vi "Get U16 Data.vi"(8 "error in (no error)":errorcluster, 11 "Data in":string) -> (0 "error out":errorcluster, 2 "U16":u16, 3 "Data out":string)   [LabVIEW 2013, in "Hierarchy Framework.lvlib" / "Section.lvclass"]
uses:
  Section.lvclass
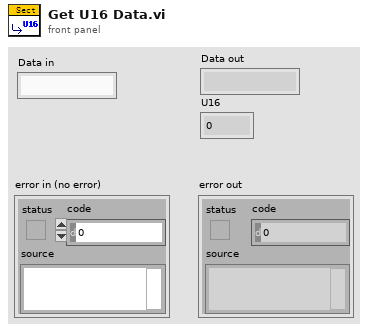
[diagram p1: front panel]
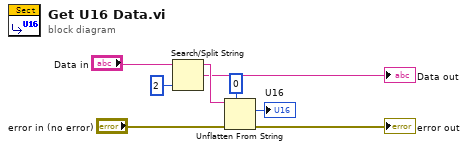
[diagram p0: block diagram]
diagram:
  n1 = Search/Split String(string="Data in", offset (0)=2 ("偏移量(0)")) -> (substring before match=w6:string, match + rest of string=→"Data out":string)  [unwired: 1 in, 1 out]
  n2 = Unflatten From String(type=u16 0 ("U16"), binary string=w6, error in (no error)="error in (no error)") -> (value=→"U16":u16, error out=→"error out":errorcluster)  [unwired: 2 in, 1 out]
